vi "addBroadcastFreezeSensorValuesFrame.vi"(8 "error in (no error)":errorcluster, 9 "BroadcastCounter":u8, 10 "ModbusBuffer in":refnum<class "ModbusBuffer.lvclass">, 11 "HPILC in":refnum<class "HPILC.lvclass">) -> (0 "error out":errorcluster, 2 "ModbusBuffer out":refnum<class "ModbusBuffer.lvclass">, 3 "HPILC out":refnum<class "HPILC.lvclass">)   [LabVIEW 2016, in "RTHPILC.lvlib" / "HPILC.lvclass"]
uses:
  HPILC.lvclass
  D:/Code/ts_M1M3Support/Common_RT_ILC/ILC/ILC.lvclass
  Common_RT_Modbus/ModbusBuffer/ModbusBuffer.lvclass
  HPILC.lvclass/HPILC.ctl
  Common_RT_ILC/ILC/ILC.lvclass/ILC.ctl
  Common_RT_Modbus/ModbusBuffer/ModbusBuffer.lvclass/ModbusBuffer.ctl
  Common_RT_Modbus/ModbusBuffer/writeByteInstruction.vi
  Common_RT_Modbus/ModbusBuffer/calculateCRC.vi
  Common_RT_ILC/ILC/ILC.lvclass
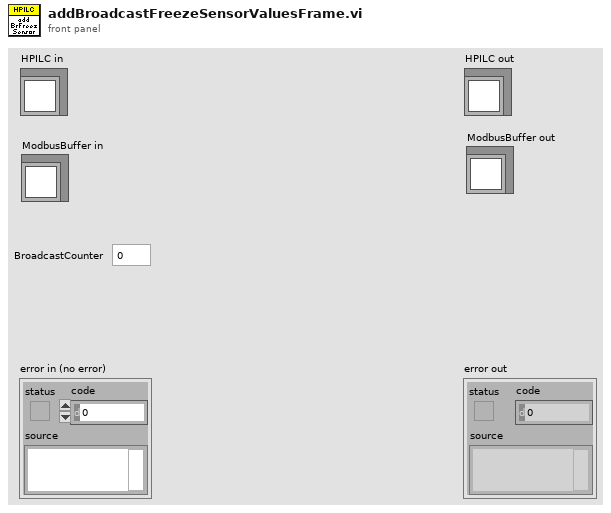
[diagram p1: front panel]
types:
  T1 = typedef "RTILC.lvlib/ILCData.ctl" = cluster{"Constants":T2, "Command":T3, "Telemetry":T5, "Responses":T6, "Timestamps":T8, "Timings":T9}
  T2 = typedef "RTILC.lvlib/ILCConstants.ctl" = cluster{"Subnet":u8, "Address":u8}
  T3 = typedef "RTILC.lvlib/ILCCommand.ctl" = cluster{"Mode":u16, "TemporaryAddress":u8, "ADCScanRate":T4, "ADCChannel":u8, "ADCOffset":sgl, "ADCSensitivity":sgl}
  T4 = typedef "RTILC.lvlib/ILCScanRates.ctl" = u8
  T5 = typedef "RTILC.lvlib/ILCTelemetry.ctl" = cluster{"UniqueID":u64, "FirmwareType":u8, "NetworkNodeType":u8, "ILCOption":u8, "NetworkNodeOption":u8, "MajorRevision":u8, "MinorRevision":u8, "FirmwareName":string, "Mode":u16, "MajorFault":bool, "MinorFault":bool, "FaultOverride":bool, "MainCalibrationError":bool, "BackupCalibrationError":bool, "UniqueIDCRCMismatch":bool, "AppTypeNodeTypeMismatch":bool, "AppMissing":bool, "AppCRCMismatch":bool, "TEDSNotFound":bool, "TEDS1Mismatch":bool, "TEDS2Mismatch":bool, "WatchdogResetDetected":bool, "BrownoutDetected":bool, "EventTrapResetDetected":bool, "MotorPowerFault":bool, "SSRPowerFault":bool, "AuxPowerFault":bool, "SMCPowerFault":bool, "TemporaryAddress":u8, "ADCScanRate":T4, "MainADCCalibrationK":sgl[], "MainSensorOffset":sgl[], "MainSensorSensitivity":sgl[], "BackupADCCalibrationK":sgl[], "BackupSensorOffset":sgl[], "BackupSensorSensitivity":sgl[]}
  T6 = typedef "RTILC.lvlib/ILCResponses.ctl" = cluster{"ReportServerID":T7, "ReportServerStatus":T7, "Mode":T7, "TemporaryAddress":T7, "Reset":T7, "ADCScanRate":T7, "ADCOffsetSensitivity":T7, "ReportCalibrationData":T7}
  T7 = typedef "RTModbus.lvlib/ExceptionCodes.ctl" = u16
  T8 = typedef "RTILC.lvlib/ILCTimestamps.ctl" = cluster{"ReportServerID":dbl, "ReportServerStatus":dbl, "Mode":dbl, "TemporaryAddress":dbl, "Reset":dbl, "ADCScanRate":dbl, "ADCOffsetSensitivity":dbl, "ReportCalibrationData":dbl}
  T9 = typedef "RTILC.lvlib/ILCTimings.ctl" = cluster{"ReportServerID":u32, "ReportServerStatus":u32, "Mode":u32, "TemporaryAddress":u32, "Reset":u32, "ADCScanRate":u32, "ADCOffsetSensitivity":u32, "ReportCalibrationData":u32}
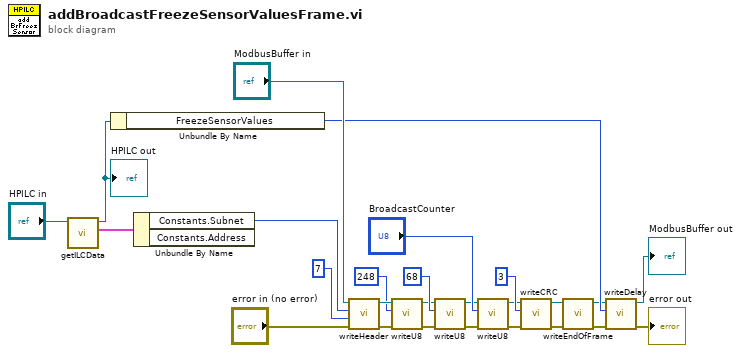
[diagram p0: block diagram]
diagram:
  n1 = call "getILCData.vi"("ILC in"="HPILC in") -> ("ILCData"=w25:T1, "ILC out"=w23:refnum<class "HPILC.lvclass">)  [unwired: 9 in]
  "HPILC out" <- w23
  n2 = Unbundle By Name(w23) -> ("FreezeSensorValues"=w15:u32)
  n3 = Unbundle By Name(w25) -> ("Constants.Subnet"=w24:u8)  [unwired: 1 out]
  n4 = call "writeHeader.vi"("error in (no error)"="error in (no error)", "Length"=u16 7, "Subnet"=w24, "ModbusBuffer in"="ModbusBuffer in") -> ("error out"=w11:errorcluster, "ModbusBuffer out"=w20:refnum<class "ModbusBuffer.lvclass">)  [unwired: 6 in]
  n5 = call "writeU8.vi"("error in (no error)"=w11, "Input"=u8 248 ("Address"), "ModbusBuffer in"=w20) -> ("error out"=w12:errorcluster, "ModbusBuffer out"=w5:refnum<class "ModbusBuffer.lvclass">)  [unwired: 7 in]
  n6 = call "writeU8.vi"("error in (no error)"=w12, "Input"=u8 68 ("Function"), "ModbusBuffer in"=w5) -> ("error out"=w13:errorcluster, "ModbusBuffer out"=w6:refnum<class "ModbusBuffer.lvclass">)  [unwired: 7 in]
  n7 = call "writeU8.vi"("error in (no error)"=w13, "Input"="BroadcastCounter", "ModbusBuffer in"=w6) -> ("error out"=w14:errorcluster, "ModbusBuffer out"=w7:refnum<class "ModbusBuffer.lvclass">)  [unwired: 7 in]
  n8 = call "writeCRC.vi"("error in (no error)"=w14, "Length"=3, "ModbusBuffer in"=w7) -> ("error out"=w1:errorcluster, "ModbusBuffer out"=w4:refnum<class "ModbusBuffer.lvclass">)  [unwired: 7 in]
  n9 = call "writeEndOfFrame.vi"("error in (no error)"=w1, "ModbusBuffer in"=w4) -> ("error out"=w2:errorcluster, "ModbusBuffer out"=w3:refnum<class "ModbusBuffer.lvclass">)  [unwired: 8 in]
  n10 = call "writeDelay.vi"("error in (no error)"=w2, "Delay(us)"=w15, "ModbusBuffer in"=w3) -> ("error out"=→"error out":errorcluster, "ModbusBuffer out"=→"ModbusBuffer out":refnum<class "ModbusBuffer.lvclass">)  [unwired: 7 in]
